vi "Check Status.vi"(8 "error in (no error)":errorcluster, 11 "Laser Power Controller in":refnum<class "Laser Power Controller.lvclass">) -> (0 "error out":errorcluster, 1 "Status":string, 2 "Ready?":bool, 3 "Laser Power Controller out":refnum<class "Laser Power Controller.lvclass">)   [LabVIEW 2009, in "Laser Power Controller.lvclass"]
doc: "(Dynamic) Check if the instrument is powered on and update its member fields with the instrument's current status. Optionally return a text status message."
uses:
  Laser Power Controller.lvclass
  Utility Classes/Scannable/Scannable.lvclass
  BEOC LPC/BEOC LPC.lvlib
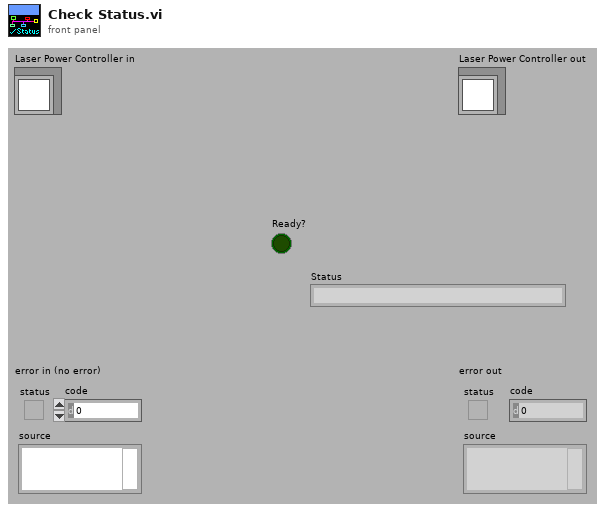
[diagram p1: front panel]
types:
  T1 = enum16{"constant power", "constant transmission"}
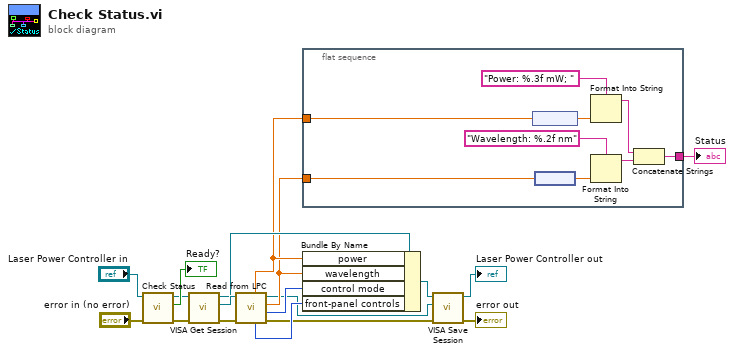
[diagram p0: block diagram]
diagram:
  n1 = call-parent "Check Status.vi"("error in (no error)"="error in (no error)", "Instrument in"="Laser Power Controller in") -> ("error out"=w6:errorcluster, "Ready?"=→"Ready?":bool, "Instrument out"=w15:refnum<class "Laser Power Controller.lvclass">)  [unwired: 6 in, 1 out]
  n2 = call-dynamic "VISA Get Session.vi"("error in (no error)"=w6, "Instrument.lvclass in"=w15) -> ("error out"=w8:errorcluster, "VISA Resource Name"=w13:refnum<visa-resource-name>, "Instrument.lvclass out"=w12:refnum<class "Laser Power Controller.lvclass">)  [unwired: 7 out]
  n3 = call "Read from LPC.vi"("error in (no error)"=w8, "VISA resource name"=w13) -> ("error out"=w7:errorcluster, "control mode"=w10:T1, "wavelength"=w3:dbl[unit], "VISA resource name out"=w1:refnum<visa-resource-name>, "front-panel controls"=w9:enum16{"enabled", "disabled"}, "power"=w4:dbl[unit])  [unwired: 4 in]
  n4 = flat-sequence {
    tunnel: w4 -> [w27]
    tunnel: w3 -> [w25]
    tunnel: [w21] -> w2
    frame #0 {
      n5 = node(w27) -> (w20:dbl)
      n6 = node(w25) -> (w19:dbl)
      n7 = Format Into String(format string="Power: %.3f mW; ", w20) -> (resulting string=w22:string)  [unwired: 2 in, 1 out]
      n8 = Format Into String(format string="Wavelength: %.2f nm", w19) -> (resulting string=w23:string)  [unwired: 2 in, 1 out]
      n9 = Concatenate Strings(w22, w23) -> (w21:string)
    }
  }
  n10 = Bundle By Name(cluster=w12, "power"=w4, "wavelength"=w3, "control mode"=w10, "front-panel controls"=w9) -> (w11:refnum<class "Laser Power Controller.lvclass">)
  n11 = call-dynamic "VISA Save Session.vi"("error in (no error)"=w7, "VISA Resource Name"=w1, "Instrument.lvclass in"=w11) -> ("error out"=→"error out":errorcluster, "Instrument.lvclass out"=→"Laser Power Controller out":refnum<class "Laser Power Controller.lvclass">)  [unwired: 7 out]
  "Status" <- w2
